vi "parse_Transform.vi"(4 "error in":errorcluster, 7 "msg in":string) -> (0 "error out":errorcluster, 2 "Transform":T1, 3 "msg out":string)   [LabVIEW 2015]
doc: "Parses a message into a transform"
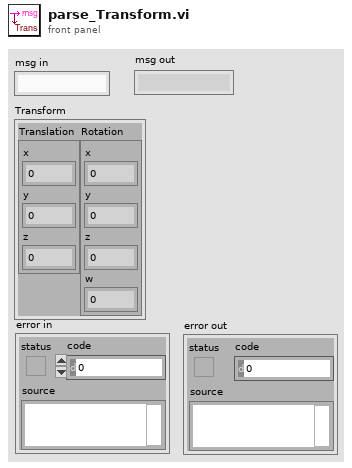
[diagram p1: front panel]
types:
  T1 = cluster{"Translation":cluster{"x":dbl, "y":dbl, "z":dbl}, "Rotation":cluster{"x":dbl, "y":dbl, "z":dbl, "w":dbl}}
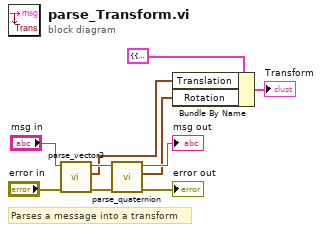
[diagram p0: block diagram]
diagram:
  # "Parses a message into a transform"
  n1 = call "parse_vector3.vi"("error in"="error in", "msg in"="msg in") -> ("error out"=w5:errorcluster, "Vector3"=w6:cluster{"x":dbl, "y":dbl, "z":dbl}, "msg out"=w7:string)  [unwired: 3 in]
  n2 = call "parse_quaternion.vi"("error in"=w5, "msg in"=w7) -> ("error out"=→"error out":errorcluster, "Quaternion"=w3:cluster{"x":dbl, "y":dbl, "z":dbl, "w":dbl}, "msg out"=→"msg out":string)  [unwired: 3 in]
  n3 = Bundle By Name(cluster=T1 {"Translation"={"x"=0.0, "y"=0.0, "z"=0.0}, "Rotation"={"x"=0.0, "y"=0.0, "z"=0.0, "w"=0.0}} ("input cluster"), "Translation"=w6, "Rotation"=w3) -> (→"Transform":T1)
